vi "Get Map PolySurf Coeffs.vi"(5 "Corrected XW map values":dbl[][](array[numeric]), 6 "surface order (n)":i32=3, 7 "cap indicial sum to n":bool) -> (0 "Ucal(m/s) coeffs":dbl[](array[numeric]), 1 "alpha(rad) coeffs":dbl[](array[numeric]), 2 "mean abs. % err in Ucal":dbl=nan format="%.6f", 3 "st. dev. in abs. % err in Ucal":dbl=-0.0 format="%.6f", 4 "coerced surface order":i32)   [LabVIEW 2010]
uses:
  XW_Map_Global.vi
  <vilib>/Analysis/Matrix/Numeric/Conversions/Array To Matrix - RA.vi
  <vilib>/Analysis/1siggen.llb/Ramp Pattern by Samples.vi
  <vilib>/Analysis/Matrix/Numeric/Conversions/Array To Matrix - RA2.vi
  <vilib>/Analysis/7linalg.llb/Solve Linear Equations (multiple right hand).vi
  <vilib>/Analysis/Matrix/Numeric/Conversions/Matrix To Array - RM.vi
  <vilib>/Analysis/baseanly.llb/Real Dot Product.vi
  <vilib>/Analysis/Matrix/NI_Matrix.lvlib
  <vilib>/Analysis/NI_AALPro.lvlib
  <vilib>/Analysis/NI_AALBase.lvlib
  <vilib>/Analysis/baseanly.llb/Real A x B.vi
  <vilib>/Analysis/7linalg.llb/Real Transpose Matrix.vi
  <vilib>/Analysis/baseanly.llb/Real Inverse Matrix.vi
panel:
  in  "Ignore first n sets when computing errors (necessary if first set is free convection set)":i32=2
  in  "What to plot":enum16{"U", "V", "Vel. magn.", "Flow angle"}(ring)=enum."Vel. magn."
  in  "Calib surface":refnum<k7>(container)
  in  "transparency":i32(knob) scale=0.0..100.0
  in  "plot style":i32(ring)=8 items=["cwLine"=1, "cwPoint"=2, "cwLinePoint"=3, "cwHiddenLine"=4, "cwSurface"=5, "cwSurfaceLine"=6, "cwSurfaceNormal"=7, "cwContourLine"=8, "cwSurfaceContour"=9]
  in  "xy projection":bool
  in  "xz projection":bool
  in  "yz projection":bool
  in  "show projections only":bool
  in  "Min. ext. fact.":dbl=1.0
  in  "Max. ext. fact.":dbl=1.0
  in  "Plot pts":i32=64
  out "min abs. % err in Ucal":dbl
  out "max abs. % err in Ucal":dbl
  out "Num. coeffs":i32
  out "Num. pts. (L)":i32
  out "Bivariate polynomial equation\n(without coeffs.)":string=" + E1^0E2^0"
  # "Paul Nathan 02/02/10"
  # "capped"
  # "not capped"
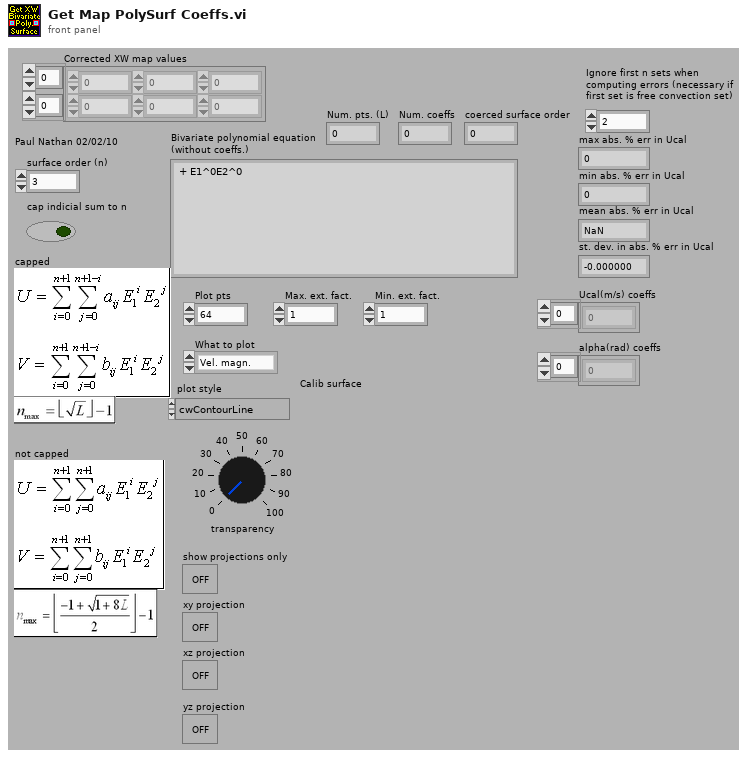
[diagram p1: front panel]
types:
  T1 = typedef "NI_Matrix.lvlib/RealMatrix.ctl" = dbl[][]
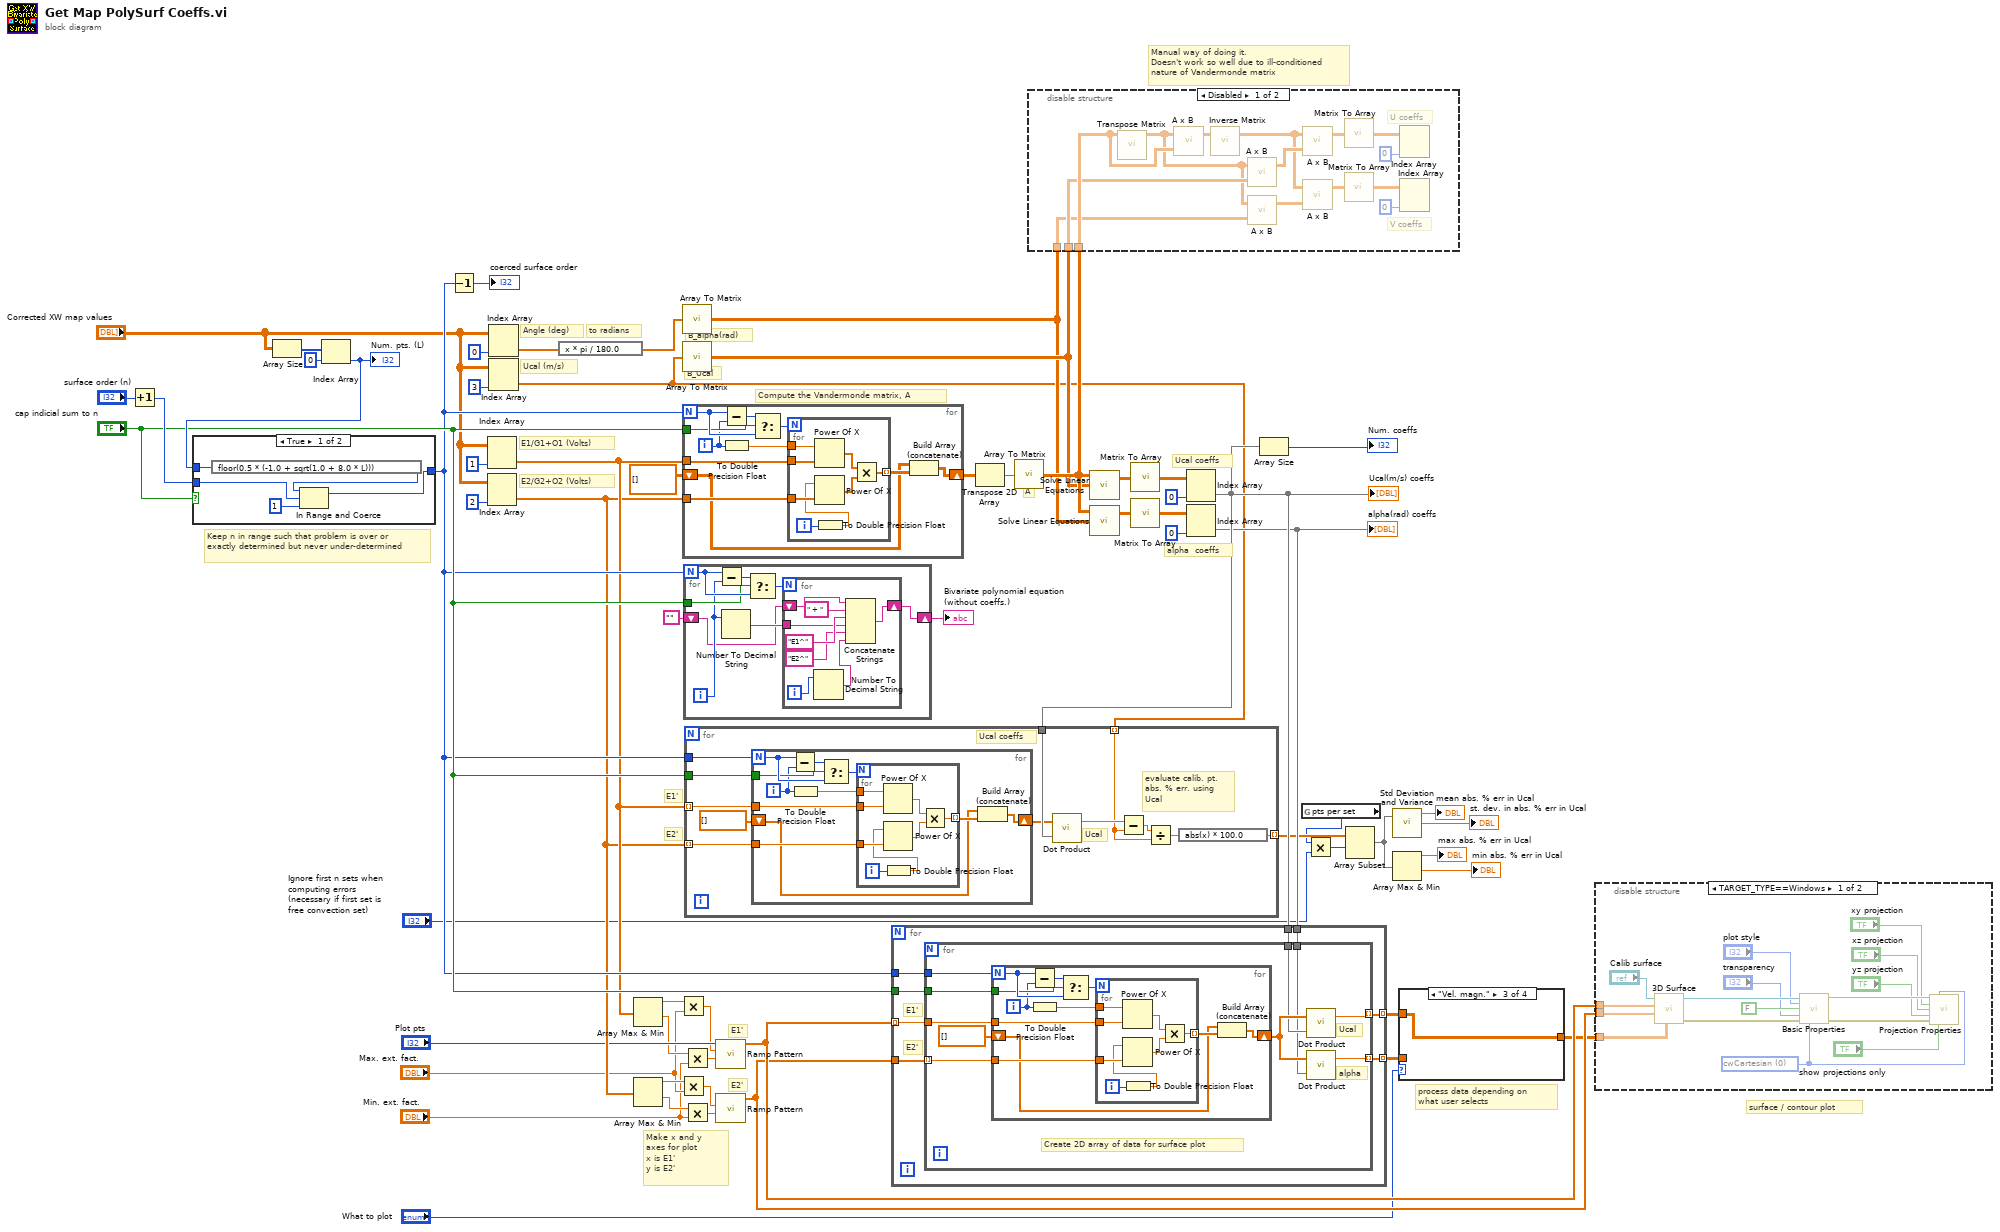
[diagram p0: block diagram]
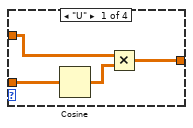
[diagram p3: hidden frame]
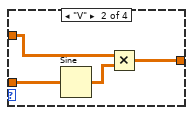
[diagram p4: hidden frame]
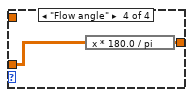
[diagram p5: hidden frame]
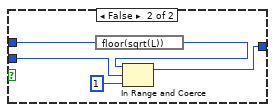
[diagram p7: hidden frame]
diagram:
  # "surface / contour plot"
  # "Make x and y axes for plot\nx is E1'\ny is E2'"
  # "process data depending on\nwhat user selects"
  # "Keep n in range such that problem is over or exactly determined but never under-determined"
  # "Manual way of doing it.\nDoesn't work so well due to ill-conditioned nature of Vandermonde matrix"
  # "E2'"
  # "E1'"
  # "E2'"
  # "E1'"
  # "alpha  coeffs"
  # "Ucal coeffs"
  # "Compute the Vandermonde matrix, A"
  # "B_alpha(rad)"
  # "B_Ucal"
  # "A"
  # "to radians"
  # "Ucal (m/s)"
  # "E2/G2+O2 (Volts)"
  # "E1/G1+O1 (Volts)"
  # "Angle (deg)"
  n1 = Increment(x="surface order (n)") -> (x+1=w38:i32)
  n2 = Array Size(array="Corrected XW map values") -> (size(s)=w46:i32[])
  n3 = Index Array(array=w46, index=0) -> (element=w37:i32)
  "Num. pts. (L)" <- w37
  n4 = case shown="True" "cap indicial sum to n" {
    tunnel: w38 -> [w63 w68]
    tunnel: [w62 w67] -> w34
    tunnel: w37 -> [w66 w71]
    frame True {
      n5 = expression code="floor(0.5 * (-1.0 + sqrt(1.0 + 8.0 * L)))"(w66) -> (w64:i32)
      n6 = In Range and Coerce(upper limit=w64, x=w63, lower limit=1 ("index")) -> (coerced(x)=w62:i32)  [unwired: 1 out]
    }
    frame False {
      n7 = expression code="floor(sqrt(L))"(w71) -> (w69:i32)
      n8 = In Range and Coerce(upper limit=w69, x=w68, lower limit=1 ("index")) -> (coerced(x)=w67:i32)  [unwired: 1 out]
    }
  }
  n9 = Decrement(x=w34) -> (x-1=→"coerced surface order":i32)
  n10 = Index Array(array="Corrected XW map values", index (col)=1 ("disabled index (col)")) -> (element=w33:dbl[])  [unwired: 1 in]
  n11 = Index Array(array="Corrected XW map values", index (col)=2 ("disabled index (col)")) -> (element=w32:dbl[])  [unwired: 1 in]
  n12 = Index Array(array="Corrected XW map values", index (col)=0 ("disabled index (col)")) -> (element=w57:dbl[])  [unwired: 1 in]
  n13 = Index Array(array="Corrected XW map values", index (col)=3 ("disabled index (col)")) -> (element=w1:dbl[])  [unwired: 1 in]
  n14 = expression code="x * pi / 180.0"(w57) -> (w2:dbl[])
  n15 = Array Max & Min(array=w33) -> (max value=w29:dbl, min value=w28:dbl)  [unwired: 2 out]
  n16 = Array Max & Min(array=w32) -> (max value=w26:dbl, min value=w22:dbl)  [unwired: 2 out]
  n17 = Multiply(x=w29, y="Max. ext. fact.") -> (x*y=w30:dbl)
  n18 = Multiply(x=w26, y="Max. ext. fact.") -> (x*y=w24:dbl)
  n19 = call-poly <vilib>:"Array To Matrix.vi"("Real 1D Array"=w2) -> ("Real Matrix (Column Vector)"=w16:T1)
  n20 = call-poly <vilib>:"Array To Matrix.vi"("Real 1D Array"=w1) -> ("Real Matrix (Column Vector)"=w17:T1)
  n21 = for {
    N: w34 -> [w81]
    tunnel: "cap indicial sum to n" -> [w80]
    tunnel: w33 -> [w78]
    tunnel: w32 -> [w77]
    shift-right: [w73] -> w54
    shift-left: dbl[][] [] -> [w72]
    i -> [w76]
    n22 = Subtract(x=w81, y=w76) -> (x-y=w82:i32)
    n23 = To Double Precision Float(number=w76) -> (double precision float=w75:dbl)
    n24 = Select(t=w82, s=w80, f=w81) -> (s? t:f=w79:i32)
    n25 = for {
      N: w79 -> [_]
      tunnel: w78 -> [w88]
      tunnel: w77 -> [w87]
      tunnel: w75 -> [w89]
      tunnel: [w83] -> w74 mode=indexing
      i -> [w90]
      # "j"
      n26 = Power Of X(1:w88, 2:w89) -> (0:w86:dbl[])
      n27 = To Double Precision Float(number=w90) -> (double precision float=w84:dbl)
      n28 = Power Of X(1:w87, 2:w84) -> (0:w85:dbl[])
      n29 = Multiply(x=w86, y=w85) -> (x*y=w83:dbl[])
    }
    n30 = Build Array (concatenate)(w72, w74) -> (w73:dbl[][])
  }
  n31 = Multiply(x=w28, y="Min. ext. fact.") -> (x*y=w27:dbl)
  n32 = Multiply(x=w22, y="Min. ext. fact.") -> (x*y=w23:dbl)
  n33 = for {
    N: w34 -> [w97]
    tunnel: "cap indicial sum to n" -> [w96]
    shift-right: [w92] -> w52
    shift-left: "" -> [w91]
    i -> [w94]
    n34 = Subtract(x=w97, y=w94) -> (x-y=w98:i32)
    n35 = Number To Decimal String(number=w94) -> (decimal integer string=w93:string)  [unwired: 1 out]
    n36 = Select(t=w98, s=w96, f=w97) -> (s? t:f=w95:i32)
    n37 = for {
      N: w95 -> [_]
      shift-right: [w105] -> w92
      shift-left: w91 -> [w104]
      tunnel: w93 -> [w101]
      i -> [w106]
      # "j"
      n38 = Number To Decimal String(number=w106) -> (decimal integer string=w99:string)  [unwired: 1 out]
      n39 = Concatenate Strings(w104, " + ", "E1^", w101, "E2^", w99) -> (w105:string)
    }
  }
  "Bivariate polynomial equation\n(without coeffs.)" <- w52
  n40 = call-poly <vilib>:"Ramp Pattern.vi"("start"=w27, "end"=w30, "samples"="Plot pts") -> ("Ramp Pattern"=w20:dbl[])  [unwired: 7 in, 1 out]
  n41 = call-poly <vilib>:"Ramp Pattern.vi"("start"=w23, "end"=w24) -> ("Ramp Pattern"=w19:dbl[])  [unwired: 8 in, 1 out]
  n42 = Transpose 2D Array(2D array=w54) -> (transposed array=w53:dbl[][])
  n43 = call-poly <vilib>:"Array To Matrix.vi"("Real 2D Array"=w53) -> ("Real Matrix"=w18:T1)
  n44 = disable-structure shown="Disabled" {
    disable-tunnel: w18 -> [w120 _]
    disable-tunnel: w17 -> [w117 _]
    disable-tunnel: w16 -> [w113 _]
    frame Disabled {
      # "V coeffs"
      # "U coeffs"
      n45 = call-poly <vilib>:"Transpose Matrix.vi"("Input Matrix"=w120) -> ("Matrix Transpose"=w114:T1)  [unwired: 10 out]
      n46 = call-poly <vilib>:"A x B.vi"("B"=w120, "A"=w114) -> ("A x B"=w119:T1)  [unwired: 1 out]
      n47 = call-poly <vilib>:"Inverse Matrix.vi"("Input Matrix"=w119) -> ("Inverse Matrix"=w116:T1)  [unwired: 1 in, 1 out]
      n48 = call-poly <vilib>:"A x B.vi"("B"=w117, "A"=w114) -> ("A x B"=w118:T1)  [unwired: 1 out]
      n49 = call-poly <vilib>:"A x B.vi"("B"=w113, "A"=w114) -> ("A x B"=w115:T1)  [unwired: 1 out]
      n50 = call-poly <vilib>:"A x B.vi"("B"=w118, "A"=w116) -> ("A x B"=w108:T1)  [unwired: 1 out]
      n51 = call-poly <vilib>:"A x B.vi"("B"=w115, "A"=w116) -> ("A x B"=w107:T1)  [unwired: 1 out]
      n52 = call-poly <vilib>:"Matrix To Array.vi"("Real Matrix"=w108) -> ("Real 2D Array"=w109:dbl[][])
      n53 = call-poly <vilib>:"Matrix To Array.vi"("Real Matrix"=w107) -> ("Real 2D Array"=w111:dbl[][])
      n54 = Index Array(array=w109, index (col)=0 ("disabled index (col)")) -> ()  [unwired: 1 in, 1 out]
      n55 = Index Array(array=w111, index (col)=0 ("disabled index (col)")) -> ()  [unwired: 1 in, 1 out]
    }
    frame Enabled {
    }
  }
  n56 = call-poly <vilib>:"Solve Linear Equations.vi"("Known Matrix"=w17, "Input Matrix"=w18) -> ("Solution Matrix"=w42:T1)  [unwired: 1 in, 1 out]
  n57 = call-poly <vilib>:"Solve Linear Equations.vi"("Known Matrix"=w16, "Input Matrix"=w18) -> ("Solution Matrix"=w41:T1)  [unwired: 1 in, 1 out]
  n58 = call-poly <vilib>:"Matrix To Array.vi"("Real Matrix"=w42) -> ("Real 2D Array"=w50:dbl[][])
  n59 = call-poly <vilib>:"Matrix To Array.vi"("Real Matrix"=w41) -> ("Real 2D Array"=w48:dbl[][])
  n60 = Index Array(array=w50, index (col)=0 ("disabled index (col)")) -> (element=w15:dbl[])  [unwired: 1 in]
  "Ucal(m/s) coeffs" <- w15
  n61 = for {
    tunnel: "cap indicial sum to n" -> [w131]
    tunnel: w34 -> [w130]
    tunnel: w15 -> [w129]
    tunnel: w33 -> [w128] mode=indexing
    tunnel: w32 -> [w127] mode=indexing
    tunnel: [w123] -> w7 mode=indexing
    tunnel: w1 -> [w121] mode=indexing
    # "evaluate calib. pt. abs. % err. using Ucal"
    # "Ucal coeffs"
    # "Ucal"
    n62 = for {
      N: w130 -> [w142]
      tunnel: w131 -> [w141]
      tunnel: w128 -> [w139]
      tunnel: w127 -> [w138]
      shift-right: [w134] -> w126
      shift-left: dbl[] [] -> [w133]
      i -> [w137]
      n63 = Subtract(x=w142, y=w137) -> (x-y=w143:i32)
      n64 = To Double Precision Float(number=w137) -> (double precision float=w136:dbl)
      n65 = Select(t=w143, s=w141, f=w142) -> (s? t:f=w140:i32)
      n66 = for {
        N: w140 -> [_]
        tunnel: w139 -> [w149]
        tunnel: w138 -> [w148]
        tunnel: w136 -> [w150]
        tunnel: [w144] -> w135 mode=indexing
        i -> [w151]
        # "j"
        n67 = Power Of X(1:w149, 2:w150) -> (0:w147:dbl)
        n68 = To Double Precision Float(number=w151) -> (double precision float=w145:dbl)
        n69 = Power Of X(1:w148, 2:w145) -> (0:w146:dbl)
        n70 = Multiply(x=w147, y=w146) -> (x*y=w144:dbl)
      }
      n71 = Build Array (concatenate)(w133, w135) -> (w134:dbl[])
    }
    n72 = call-poly <vilib>:"Dot Product.vi"("Y Vector"=w129, "X Vector"=w126) -> ("X * Y"=w122:dbl)  [unwired: 1 out]
    n73 = Subtract(x=w122, y=w121) -> (x-y=w125:dbl)
    n74 = Divide(x=w125, y=w121) -> (x/y=w124:dbl)
    n75 = expression code="abs(x) * 100.0"(w124) -> (w123:dbl)
  }
  n76 = Index Array(array=w48, index (col)=0 ("disabled index (col)")) -> (element=w14:dbl[])  [unwired: 1 in]
  "alpha(rad) coeffs" <- w14
  n77 = for {
    tunnel: "cap indicial sum to n" -> [w159]
    tunnel: w34 -> [w158]
    tunnel: w20 -> [w157] mode=indexing
    tunnel: w19 -> [w156]
    tunnel: w15 -> [w155]
    tunnel: w14 -> [w154]
    tunnel: [w153] -> w11 mode=indexing
    tunnel: [w152] -> w10 mode=indexing
    # "E2'"
    # "E1'"
    n78 = for {
      tunnel: w159 -> [w168]
      tunnel: w158 -> [w167]
      tunnel: w157 -> [w166]
      tunnel: w156 -> [w165] mode=indexing
      tunnel: [w163] -> w153 mode=indexing
      tunnel: [w162] -> w152 mode=indexing
      tunnel: w155 -> [w161]
      tunnel: w154 -> [w160]
      # "Create 2D array of data for surface plot"
      # "alpha"
      # "Ucal"
      n79 = for {
        N: w167 -> [w179]
        tunnel: w168 -> [w178]
        tunnel: w166 -> [w176]
        tunnel: w165 -> [w175]
        shift-right: [w171] -> w164
        shift-left: dbl[] [] -> [w170]
        i -> [w174]
        n80 = Subtract(x=w179, y=w174) -> (x-y=w180:i32)
        n81 = To Double Precision Float(number=w174) -> (double precision float=w173:dbl)
        n82 = Select(t=w180, s=w178, f=w179) -> (s? t:f=w177:i32)
        n83 = for {
          N: w177 -> [_]
          tunnel: w176 -> [w186]
          tunnel: w175 -> [w185]
          tunnel: w173 -> [w187]
          tunnel: [w181] -> w172 mode=indexing
          i -> [w188]
          # "j"
          n84 = Power Of X(1:w186, 2:w187) -> (0:w184:dbl)
          n85 = To Double Precision Float(number=w188) -> (double precision float=w182:dbl)
          n86 = Power Of X(1:w185, 2:w182) -> (0:w183:dbl)
          n87 = Multiply(x=w184, y=w183) -> (x*y=w181:dbl)
        }
        n88 = Build Array (concatenate)(w170, w172) -> (w171:dbl[])
      }
      n89 = call-poly <vilib>:"Dot Product.vi"("Y Vector"=w161, "X Vector"=w164) -> ("X * Y"=w163:dbl)  [unwired: 1 out]
      n90 = call-poly <vilib>:"Dot Product.vi"("Y Vector"=w160, "X Vector"=w164) -> ("X * Y"=w162:dbl)  [unwired: 1 out]
    }
  }
  n91 = Array Size(array=w15) -> (size(s)=→"Num. coeffs":i32)
  n92 = global read "XW_Map_Global.vi" "pts per set"() -> (w3:i32)
  n93 = Multiply(x=w3, y="Ignore first n sets when computing errors (necessary if first set is free convection set)") -> (x*y=w5:i32)
  n94 = Array Subset(array=w7, index=w5) -> (w6:dbl[])  [unwired: 1 in]
  n95 = call <vilib>:"Std Deviation and Variance.vi"("X"=w6) -> ("mean"=→"mean abs. % err in Ucal":dbl, "standard deviation"=→"st. dev. in abs. % err in Ucal":dbl)  [unwired: 1 in, 1 out]
  n96 = Array Max & Min(array=w6) -> (max value=→"max abs. % err in Ucal":dbl, min value=→"min abs. % err in Ucal":dbl)  [unwired: 2 out]
  n97 = case shown="\"Vel. magn.\"" "What to plot" {
    tunnel: [w189 w196 w197 w199] -> w12
    tunnel: w11 -> [w191 w195 w197 _]
    tunnel: w10 -> [w192 w193 _ w198]
    frame "U" {
      n98 = Cosine(x=w192) -> (cos(x)=w190:dbl[][])
      n99 = Multiply(x=w191, y=w190) -> (x*y=w189:dbl[][])
    }
    frame "V" {
      n100 = Sine(x=w193) -> (sin(x)=w194:dbl[][])
      n101 = Multiply(x=w195, y=w194) -> (x*y=w196:dbl[][])
    }
    frame "Vel. magn." {
    }
    frame "Flow angle" {
      n102 = expression code="x * 180.0 / pi"(w198) -> (w199:dbl[][])
    }
  }
  n103 = disable-structure shown="TARGET_TYPE==Windows" {
    disable-tunnel: w20 -> [w215 _]
    disable-tunnel: w19 -> [w214 _]
    disable-tunnel: w12 -> [w213 _]
    frame condition #0 {
      w206 = 0 items=["cwCartesian", "cwCylindrical", "cwSpherical"] ("coordinate system")
      n104 = call <vilib>:"3D Surface.vi"("z matrix"=w213, "y vector"=w214, "x vector"=w215, "3D graph"="Calib surface") -> ("error out"=w210:errorcluster, "3D graph out"=w211:refnum<k7>)  [unwired: 1 in, 5 out]
      n105 = call <vilib>:"Basic Properties.vi"("3D graph"=w211, "plot style"="plot style", "fast draw"=FALSE, "transparency"="transparency", "error in (no error)"=w210, "coordinate system"=w206) -> ("3D graph out"=w209:refnum<k7>, "error out"=w208:errorcluster)  [unwired: 8 out]
      n106 = call <vilib>:"Projection Properties.vi"("3D graph"=w209, "coordinate system"=w206, "xy projection"="xy projection", "xz projection"="xz projection", "yz projection"="yz projection", "error in (no error)"=w208, "show projections only"="show projections only") -> ()  [unwired: 1 in, 8 out]
    }
    frame condition #1 (active) {
    }
  }
